vi "Test - Draw Teapot.vi"() -> ()   [LabVIEW 2022 SP3, in "Raster.lvlib"] (continued)
"v"=0.0}, "Colour"=12517256}, "Vertex 3"={"Position"={"x"=109.02176, "y"=274.10672, "z"=0.98959744}, "UV"={"u"=0.0, "v"=0.0}, "Colour"=12517256}, "Alpha"=0.0, "Alpha Blending Enabled"=FALSE, "Colour"=9684586}, {"Vertex 1"={"Position"={"x"=98.163345, "y"=283.49265, "z"=0.9895778}, "UV"={"u"=0.0, "v"=0.0}, "Colour"=12517256}, "Vertex 2"={"Position"={"x"=104.74968, "y"=271.31357, "z"=0.9895778}, "UV"={"u"=0.0, "v"=0.0}, "Colour"=12517256}, "Vertex 3"={"Position"={"x"=101.588585, "y"=268.6284, "z"=0.98959744}, "UV"={"u"=0.0, "v"=0.0}, "Colour"=12517256}, "Alpha"=0.0, "Alpha Blending Enabled"=FALSE, "Colour"=7773780}, {"Vertex 1"={"Position"={"x"=104.74968, "y"=271.31357, "z"=0.9895778}, "UV"={"u"=0.0, "v"=0.0}, "Colour"=12517256}, "Vertex 2"={"Position"={"x"=98.163345, "y"=283.49265, "z"=0.9895778}, "UV"={"u"=0.0, "v"=0.0}, "Colour"=12517256}, "Vertex 3"={"Position"={"x"=102.92444, "y"=285.8186, "z"=0.98959744}, "UV"={"u"=0.0, "v"=0.0}, "Colour"=12517256}, "Alpha"=0.0, "Alpha Blending Enabled"=FALSE, "Colour"=9486951}, {"Vertex 1"={"Position"={"x"=93.51947, "y"=295.5369, "z"=0.9895778}, "UV"={"u"=0.0, "v"=0.0}, "Colour"=12517256}, "Vertex 2"={"Position"={"x"=98.163345, "y"=283.49265, "z"=0.9895778}, "UV"={"u"=0.0, "v"=0.0}, "Colour"=12517256}, "Vertex 3"={"Position"={"x"=94.53805, "y"=281.22873, "z"=0.98959744}, "UV"={"u"=0.0, "v"=0.0}, "Colour"=12517256}, "Alpha"=0.0, "Alpha Blending Enabled"=FALSE, "Colour"=8037207}, {"Vertex 1"={"Position"={"x"=98.163345, "y"=283.49265, "z"=0.9895778}, "UV"={"u"=0.0, "v"=0.0}, "Colour"=12517256}, "Vertex 2"={"Position"={"x"=93.51947, "y"=295.5369, "z"=0.9895778}, "UV"={"u"=0.0, "v"=0.0}, "Colour"=12517256}, "Vertex 3"={"Position"={"x"=98.63565, "y"=297.2621, "z"=0.98959744}, "UV"={"u"=0.0, "v"=0.0}, "Colour"=12517256}, "Alpha"=0.0, "Alpha Blending Enabled"=FALSE, "Colour"=9289317}, {"Vertex 1"={"Position"={"x"=90.76903, "y"=307.28738, "z"=0.9895778}, "UV"={"u"=0.0, "v"=0.0}, "Colour"=12517256}, "Vertex 2"={"Position"={"x"=93.51947, "y"=295.5369, "z"=0.9895778}, "UV"={"u"=0.0, "v"=0.0}, "Colour"=12517256}, "Vertex 3"={"Position"={"x"=89.5565, "y"=293.82855, "z"=0.98959744}, "UV"={"u"=0.0, "v"=0.0}, "Colour"=12517256}, "Alpha"=0.0, "Alpha Blending Enabled"=FALSE, "Colour"=8300890}, {"Vertex 1"={"Position"={"x"=93.51947, "y"=295.5369, "z"=0.9895778}, "UV"={"u"=0.0, "v"=0.0}, "Colour"=12517256}, "Vertex 2"={"Position"={"x"=90.76903, "y"=307.28738, "z"=0.9895778}, "UV"={"u"=0.0, "v"=0.0}, "Colour"=12517256}, "Vertex 3"={"Position"={"x"=96.10178, "y"=308.23883, "z"=0.98959744}, "UV"={"u"=0.0, "v"=0.0}, "Colour"=12517256}, "Alpha"=0.0, "Alpha Blending Enabled"=FALSE, "Colour"=9091427}, {"Vertex 1"={"Position"={"x"=89.86314, "y"=318.58496, "z"=0.9895778}, "UV"={"u"=0.0, "v"=0.0}, "Colour"=12517256}, "Vertex 2"={"Position"={"x"=90.76903, "y"=307.28738, "z"=0.9895778}, "UV"={"u"=0.0, "v"=0.0}, "Colour"=12517256}, "Vertex 3"={"Position"={"x"=86.5999, "y"=306.30865, "z"=0.98959744}, "UV"={"u"=0.0, "v"=0.0}, "Colour"=12517256}, "Alpha"=0.0, "Alpha Blending Enabled"=FALSE, "Colour"=8564317}, {"Vertex 1"={"Position"={"x"=90.76903, "y"=307.28738, "z"=0.9895778}, "UV"={"u"=0.0, "v"=0.0}, "Colour"=12517256}, "Vertex 2"={"Position"={"x"=89.86314, "y"=318.58496, "z"=0.9895778}, "UV"={"u"=0.0, "v"=0.0}, "Colour"=12517256}, "Vertex 3"={"Position"={"x"=95.26916, "y"=318.55002, "z"=0.98959744}, "UV"={"u"=0.0, "v"=0.0}, "Colour"=12517256}, "Alpha"=0.0, "Alpha Blending Enabled"=FALSE, "Colour"=8828000}, {"Vertex 1"={"Position"={"x"=91.32674, "y"=328.538, "z"=0.9895778}, "UV"={"u"=0.0, "v"=0.0}, "Colour"=12517256}, "Vertex 2"={"Position"={"x"=89.86314, "y"=318.58496, "z"=0.9895778}, "UV"={"u"=0.0, "v"=0.0}, "Colour"=12517256}, "Vertex 3"={"Position"={"x"=85.62412, "y"=318.55002, "z"=0.98959744}, "UV"={"u"=0.0, "v"=0.0}, "Colour"=12517256}, "Alpha"=0.0, "Alpha Blending Enabled"=FALSE, "Colour"=8959585}, {"Vertex 1"={"Position"={"x"=89.86314, "y"=318.58496, "z"=0.9895778}, "UV"={"u"=0.0, "v"=0.0}, "Colour"=12517256}, "Vertex 2"={"Position"={"x"=91.32674, "y"=328.538, "z"=0.9895778}, "UV"={"u"=0.0, "v"=0.0}, "Colour"=12517256}, "Vertex 3"={"Position"={"x"=96.68016, "y"=327.50403, "z"=0.98959744}, "UV"={"u"=0.0, "v"=0.0}, "Colour"=12517256}, "Alpha"=0.0, "Alpha Blending Enabled"=FALSE, "Colour"=8432732}, {"Vertex 1"={"Position"={"x"=95.695854, "y"=336.50763, "z"=0.9895778}, "UV"={"u"=0.0, "v"=0.0}, "Colour"=12517256}, "Vertex 2"={"Position"={"x"=91.32674, "y"=328.538, "z"=0.9895778}, "UV"={"u"=0.0, "v"=0.0}, "Colour"=12517256}, "Vertex 3"={"Position"={"x"=87.13484, "y"=329.46445, "z"=0.98959744}, "UV"={"u"=0.0, "v"=0.0}, "Colour"=12517256}, "Alpha"=0.0, "Alpha Blending Enabled"=FALSE, "Colour"=9552488}, {"Vertex 1"={"Position"={"x"=91.32674, "y"=328.538, "z"=0.9895778}, "UV"={"u"=0.0, "v"=0.0}, "Colour"=12517256}, "Vertex 2"={"Position"={"x"=95.695854, "y"=336.50763, "z"=0.9895778}, "UV"={"u"=0.0, "v"=0.0}, "Colour"=12517256}, "Vertex 3"={"Position"={"x"=100.88518, "y"=334.67392, "z"=0.98959744}, "UV"={"u"=0.0, "v"=0.0}, "Colour"=12517256}, "Alpha"=0.0, "Alpha Blending Enabled"=FALSE, "Colour"=7839829}, {"Vertex 1"={"Position"={"x"=102.93782, "y"=342.71442, "z"=0.9895778}, "UV"={"u"=0.0, "v"=0.0}, "Colour"=12517256}, "Vertex 2"={"Position"={"x"=95.695854, "y"=336.50763, "z"=0.9895778}, "UV"={"u"=0.0, "v"=0.0}, "Colour"=12517256}, "Vertex 3"={"Position"={"x"=91.65158, "y"=338.20395, "z"=0.98959744}, "UV"={"u"=0.0, "v"=0.0}, "Colour"=12517256}, "Alpha"=0.0, "Alpha Blending Enabled"=FALSE, "Colour"=10079854}, {"Vertex 1"={"Position"={"x"=95.695854, "y"=336.50763, "z"=0.9895778}, "UV"={"u"=0.0, "v"=0.0}, "Colour"=12517256}, "Vertex 2"={"Position"={"x"=102.93782, "y"=342.71442, "z"=0.9895778}, "UV"={"u"=0.0, "v"=0.0}, "Colour"=12517256}, "Vertex 3"={"Position"={"x"=107.84178, "y"=340.25775, "z"=0.98959744}, "UV"={"u"=0.0, "v"=0.0}, "Colour"=12517256}, "Alpha"=0.0, "Alpha Blending Enabled"=FALSE, "Colour"=7246927}, {"Vertex 1"={"Position"={"x"=113.01999, "y"=347.37875, "z"=0.9895778}, "UV"={"u"=0.0, "v"=0.0}, "Colour"=12517256}, "Vertex 2"={"Position"={"x"=102.93782, "y"=342.71442, "z"=0.9895778}, "UV"={"u"=0.0, "v"=0.0}, "Colour"=12517256}, "Vertex 3"={"Position"={"x"=99.15168, "y"=345.0104, "z"=0.98959744}, "UV"={"u"=0.0, "v"=0.0}, "Colour"=12517256}, "Alpha"=0.0, "Alpha Blending Enabled"=FALSE, "Colour"=10540658}, {"Vertex 1"={"Position"={"x"=102.93782, "y"=342.71442, "z"=0.9895778}, "UV"={"u"=0.0, "v"=0.0}, "Colour"=12517256}, "Vertex 2"={"Position"={"x"=113.01999, "y"=347.37875, "z"=0.9895778}, "UV"={"u"=0.0, "v"=0.0}, "Colour"=12517256}, "Vertex 3"={"Position"={"x"=117.50798, "y"=344.45398, "z"=0.98959744}, "UV"={"u"=0.0, "v"=0.0}, "Colour"=12517256}, "Alpha"=0.0, "Alpha Blending Enabled"=FALSE, "Colour"=6785866}, {"Vertex 1"={"Position"={"x"=125.90974, "y"=350.72086, "z"=0.9895778}, "UV"={"u"=0.0, "v"=0.0}, "Colour"=12517256}, "Vertex 2"={"Position"={"x"=113.01999, "y"=347.37875, "z"=0.9895778}, "UV"={"u"=0.0, "v"=0.0}, "Colour"=12517256}, "Vertex 3"={"Position"={"x"=109.61189, "y"=350.12524, "z"=0.98959744}, "UV"={"u"=0.0, "v"=0.0}, "Colour"=12517256}, "Alpha"=0.0, "Alpha Blending Enabled"=FALSE, "Colour"=10738549}, {"Vertex 1"={"Position"={"x"=113.01999, "y"=347.37875, "z"=0.9895778}, "UV"={"u"=0.0, "v"=0.0}, "Colour"=12517256}, "Vertex 2"={"Position"={"x"=125.90974, "y"=350.72086, "z"=0.9895778}, "UV"={"u"=0.0, "v"=0.0}, "Colour"=12517256}, "Vertex 3"={"Position"={"x"=129.84137, "y"=347.46066, "z"=0.98959744}, "UV"={"u"=0.0, "v"=0.0}, "Colour"=12517256}, "Alpha"=0.0, "Alpha Blending Enabled"=FALSE, "Colour"=6522183}, {"Vertex 1"={"Position"={"x"=141.57439, "y"=352.9612, "z"=0.9895778}, "UV"={"u"=0.0, "v"=0.0}, "Colour"=12517256}, "Vertex 2"={"Position"={"x"=125.90974, "y"=350.72086, "z"=0.9895778}, "UV"={"u"=0.0, "v"=0.0}, "Colour"=12517256}, "Vertex 3"={"Position"={"x"=123.00947, "y"=353.7902, "z"=0.98959744}, "UV"={"u"=0.0, "v"=0.0}, "Colour"=12517256}, "Alpha"=0.0, "Alpha Blending Enabled"=FALSE, "Colour"=10804598}, {"Vertex 1"={"Position"={"x"=125.90974, "y"=350.72086, "z"=0.9895778}, "UV"={"u"=0.0, "v"=0.0}, "Colour"=12517256}, "Vertex 2"={"Position"={"x"=141.57439, "y"=352.9612, "z"=0.9895778}, "UV"={"u"=0.0, "v"=0.0}, "Colour"=12517256}, "Vertex 3"={"Position"={"x"=144.79973, "y"=349.47617, "z"=0.98959744}, "UV"={"u"=0.0, "v"=0.0}, "Colour"=12517256}, "Alpha"=0.0, "Alpha Blending Enabled"=FALSE, "Colour"=6324549}, {"Vertex 1"={"Position"={"x"=159.98125, "y"=354.3201, "z"=0.9895778}, "UV"={"u"=0.0, "v"=0.0}, "Colour"=12517256}, "Vertex 2"={"Position"={"x"=141.57439, "y"=352.9612, "z"=0.9895778}, "UV"={"u"=0.0, "v"=0.0}, "Colour"=12517256}, "Vertex 3"={"Position"={"x"=139.3214, "y"=356.247, "z"=0.98959744}, "UV"={"u"=0.0, "v"=0.0}, "Colour"=12517256}, "Alpha"=0.0, "Alpha Blending Enabled"=FALSE, "Colour"=10870134}, {"Vertex 1"={"Position"={"x"=141.57439, "y"=352.9612, "z"=0.9895778}, "UV"={"u"=0.0, "v"=0.0}, "Colour"=12517256}, "Vertex 2"={"Position"={"x"=159.98125, "y"=354.3201, "z"=0.9895778}, "UV"={"u"=0.0, "v"=0.0}, "Colour"=12517256}, "Vertex 3"={"Position"={"x"=162.341, "y"=350.69873, "z"=0.98959744}, "UV"={"u"=0.0, "v"=0.0}, "Colour"=12517256}, "Alpha"=0.0, "Alpha Blending Enabled"=FALSE, "Colour"=6258756}, {"Vertex 1"={"Position"={"x"=181.09776, "y"=355.0179, "z"=0.9895778}, "UV"={"u"=0.0, "v"=0.0}, "Colour"=12517256}, "Vertex 2"={"Position"={"x"=159.98125, "y"=354.3201, "z"=0.9895778}, "UV"={"u"=0.0, "v"=0.0}, "Colour"=12517256}, "Vertex 3"={"Position"={"x"=158.52467, "y"=357.73706, "z"=0.98959744}, "UV"={"u"=0.0, "v"=0.0}, "Colour"=12517256}, "Alpha"=0.0, "Alpha Blending Enabled"=FALSE, "Colour"=10870134}, {"Vertex 1"={"Position"={"x"=159.98125, "y"=354.3201, "z"=0.9895778}, "UV"={"u"=0.0, "v"=0.0}, "Colour"=12517256}, "Vertex 2"={"Position"={"x"=181.09776, "y"=355.0179, "z"=0.9895778}, "UV"={"u"=0.0, "v"=0.0}, "Colour"=12517256}, "Vertex 3"={"Position"={"x"=182.42264, "y"=351.32635, "z"=0.98959744}, "UV"={"u"=0.0, "v"=0.0}, "Colour"=12517256}, "Alpha"=0.0, "Alpha Blending Enabled"=FALSE, "Colour"=6258500}, {"Vertex 1"={"Position"={"x"=204.89125, "y"=355.27502, "z"=0.9895778}, "UV"={"u"=0.0, "v"=0.0}, "Colour"=12517256}, "Vertex 2"={"Position"={"x"=181.09776, "y"=355.0179, "z"=0.9895778}, "UV"={"u"=0.0, "v"=0.0}, "Colour"=12517256}, "Vertex 3"={"Position"={"x"=180.59659, "y"=358.50238, "z"=0.98959744}, "UV"={"u"=0.0, "v"=0.0}, "Colour"=12517256}, "Alpha"=0.0, "Alpha Blending Enabled"=FALSE, "Colour"=10870134}, {"Vertex 1"={"Position"={"x"=181.09776, "y"=355.0179, "z"=0.9895778}, "UV"={"u"=0.0, "v"=0.0}, "Colour"=12517256}, "Vertex 2"={"Position"={"x"=204.89125, "y"=355.27502, "z"=0.9895778}, "UV"={"u"=0.0, "v"=0.0}, "Colour"=12517256}, "Vertex 3"={"Position"={"x"=205.00276, "y"=351.5577, "z"=0.98959744}, "UV"={"u"=0.0, "v"=0.0}, "Colour"=12517256}, "Alpha"=0.0, "Alpha Blending Enabled"=FALSE, "Colour"=6258500}, {"Vertex 1"={"Position"={"x"=231.32906, "y"=355.31174, "z"=0.9895778}, "UV"={"u"=0.0, "v"=0.0}, "Colour"=12517256}, "Vertex 2"={"Position"={"x"=204.89125, "y"=355.27502, "z"=0.9895778}, "UV"={"u"=0.0, "v"=0.0}, "Colour"=12517256}, "Vertex 3"={"Position"={"x"=205.5139, "y"=358.7842, "z"=0.98959744}, "UV"={"u"=0.0, "v"=0.0}, "Colour"=12517256}, "Alpha"=0.0, "Alpha Blending Enabled"=FALSE, "Colour"=10870134}, {"Vertex 1"={"Position"={"x"=204.89125, "y"=355.27502, "z"=0.9895778}, "UV"={"u"=0.0, "v"=0.0}, "Colour"=12517256}, "Vertex 2"={"Position"={"x"=231.32906, "y"=355.31174, "z"=0.9895778}, "UV"={"u"=0.0, "v"=0.0}, "Colour"=12517256}, "Vertex 3"={"Position"={"x"=230.03891, "y"=351.59073, "z"=0.98959744}, "UV"={"u"=0.0, "v"=0.0}, "Colour"=12517256}, "Alpha"=0.0, "Alpha Blending Enabled"=FALSE, "Colour"=6258500}, {"Vertex 1"={"Position"={"x"=583.19836, "y"=275.50385, "z"=0.9896794}, "UV"={"u"=0.0, "v"=0.0}, "Colour"=12517256}, "Vertex 2"={"Position"={"x"=608.8621, "y"=277.8157, "z"=0.9896861}, "UV"={"u"=0.0, "v"=0.0}, "Colour"=12517256}, "Vertex 3"={"Position"={"x"=615.98, "y"=270.86078, "z"=0.989385}, "UV"={"u"=0.0, "v"=0.0}, "Colour"=12517256}, "Alpha"=0.0, "Alpha Blending Enabled"=FALSE, "Colour"=11594878}, {"Vertex 1"={"Position"={"x"=689.394, "y"=356.5748, "z"=0.98960906}, "UV"={"u"=0.0, "v"=0.0}, "Colour"=12517256}, "Vertex 2"={"Position"={"x"=683.931, "y"=340.25684, "z"=0.98953646}, "UV"={"u"=0.0, "v"=0.0}, "Colour"=12517256}, "Vertex 3"={"Position"={"x"=677.0391, "y"=342.4919, "z"=0.9896034}, "UV"={"u"=0.0, "v"=0.0}, "Colour"=12517256}, "Alpha"=0.0, "Alpha Blending Enabled"=FALSE, "Colour"=10672756}, {"Vertex 1"={"Position"={"x"=180.41942, "y"=218.89479, "z"=0.9893465}, "UV"={"u"=0.0, "v"=0.0}, "Colour"=12517256}, "Vertex 2"={"Position"={"x"=182.0637, "y"=204.669, "z"=0.98935175}, "UV"={"u"=0.0, "v"=0.0}, "Colour"=12517256}, "Vertex 3"={"Position"={"x"=193.60881, "y"=210.88196, "z"=0.990049}, "UV"={"u"=0.0, "v"=0.0}, "Colour"=12517256}, "Alpha"=0.0, "Alpha Blending Enabled"=FALSE, "Colour"=131841}, {"Vertex 1"={"Position"={"x"=617.93634, "y"=204.669, "z"=0.98935175}, "UV"={"u"=0.0, "v"=0.0}, "Colour"=12517256}, "Vertex 2"={"Position"={"x"=619.58057, "y"=218.89479, "z"=0.9893465}, "UV"={"u"=0.0, "v"=0.0}, "Colour"=12517256}, "Vertex 3"={"Position"={"x"=607.8461, "y"=224.21788, "z"=0.990049}, "UV"={"u"=0.0, "v"=0.0}, "Colour"=12517256}, "Alpha"=0.0, "Alpha Blending Enabled"=FALSE, "Colour"=131841}, {"Vertex 1"={"Position"={"x"=181.27118, "y"=234.16856, "z"=0.98934925}, "UV"={"u"=0.0, "v"=0.0}, "Colour"=12517256}, "Vertex 2"={"Position"={"x"=180.41942, "y"=218.89479, "z"=0.9893465}, "UV"={"u"=0.0, "v"=0.0}, "Colour"=12517256}, "Vertex 3"={"Position"={"x"=192.15388, "y"=224.21788, "z"=0.990049}, "UV"={"u"=0.0, "v"=0.0}, "Colour"=12517256}, "Alpha"=0.0, "Alpha Blending Enabled"=FALSE, "Colour"=1185805}, {"Vertex 1"={"Position"={"x"=619.58057, "y"=218.89479, "z"=0.9893465}, "UV"={"u"=0.0, "v"=0.0}, "Colour"=12517256}, "Vertex 2"={"Position"={"x"=618.7288, "y"=234.16856, "z"=0.98934925}, "UV"={"u"=0.0, "v"=0.0}, "Colour"=12517256}, "Vertex 3"={"Position"={"x"=607.09265, "y"=238.47354, "z"=0.990049}, "UV"={"u"=0.0, "v"=0.0}, "Colour"=12517256}, "Alpha"=0.0, "Alpha Blending Enabled"=FALSE, "Colour"=1185805}, {"Vertex 1"={"Position"={"x"=389.09088, "y"=464.3185, "z"=0.98942566}, "UV"={"u"=0.0, "v"=0.0}, "Colour"=12517256}, "Vertex 2"={"Position"={"x"=393.28003, "y"=463.19003, "z"=0.98966503}, "UV"={"u"=0.0, "v"=0.0}, "Colour"=12517256}, "Vertex 3"={"Position"={"x"=396.5364, "y"=463.4357, "z"=0.9896494}, "UV"={"u"=0.0, "v"=0.0}, "Colour"=12517256}, "Alpha"=0.0, "Alpha Blending Enabled"=FALSE, "Colour"=10409073}, {"Vertex 1"={"Position"={"x"=621.5498, "y"=201.64421, "z"=0.9896861}, "UV"={"u"=0.0, "v"=0.0}, "Colour"=12517256}, "Vertex 2"={"Position"={"x"=583.19836, "y"=191.57744, "z"=0.9896794}, "UV"={"u"=0.0, "v"=0.0}, "Colour"=12517256}, "Vertex 3"={"Position"={"x"=588.6202, "y"=195.32538, "z"=0.9893725}, "UV"={"u"=0.0, "v"=0.0}, "Colour"=12517256}, "Alpha"=0.0, "Alpha Blending Enabled"=FALSE, "Colour"=131841}, {"Vertex 1"={"Position"={"x"=683.931, "y"=340.25684, "z"=0.98953646}, "UV"={"u"=0.0, "v"=0.0}, "Colour"=12517256}, "Vertex 2"={"Position"={"x"=689.394, "y"=356.5748, "z"=0.98960906}, "UV"={"u"=0.0, "v"=0.0}, "Colour"=12517256}, "Vertex 3"={"Position"={"x"=696.25714, "y"=355.18262, "z"=0.98958987}, "UV"={"u"=0.0, "v"=0.0}, "Colour"=12517256}, "Alpha"=0.0, "Alpha Blending Enabled"=FALSE, "Colour"=10738549}, {"Vertex 1"={"Position"={"x"=394.9576, "y"=413.28833, "z"=0.9894651}, "UV"={"u"=0.0, "v"=0.0}, "Colour"=12517256}, "Vertex 2"={"Position"={"x"=396.44946, "y"=415.85388, "z"=0.98963785}, "UV"={"u"=0.0, "v"=0.0}, "Colour"=12517256}, "Vertex 3"={"Position"={"x"=400.0, "y"=415.91602, "z"=0.9896323}, "UV"={"u"=0.0, "v"=0.0}, "Colour"=12517256}, "Alpha"=0.0, "Alpha Blending Enabled"=FALSE, "Colour"=11924353}, {"Vertex 1"={"Position"={"x"=400.0, "y"=130.68715, "z"=0.990049}, "UV"={"u"=0.0, "v"=0.0}, "Colour"=12517256}, "Vertex 2"={"Position"={"x"=374.42786, "y"=119.574394, "z"=0.98937833}, "UV"={"u"=0.0, "v"=0.0}, "Colour"=12517256}, "Vertex 3"={"Position"={"x"=379.93253, "y"=118.36189, "z"=0.9893066}, "UV"={"u"=0.0, "v"=0.0}, "Colour"=12517256}, "Alpha"=0.0, "Alpha Blending Enabled"=FALSE, "Colour"=131841}, {"Vertex 1"={"Position"={"x"=400.0, "y"=130.68715, "z"=0.990049}, "UV"={"u"=0.0, "v"=0.0}, "Colour"=12517256}, "Vertex 2"={"Position"={"x"=420.06744, "y"=118.36189, "z"=0.9893066}, "UV"={"u"=0.0, "v"=0.0}, "Colour"=12517256}, "Vertex 3"={"Position"={"x"=425.57214, "y"=119.574394, "z"=0.98937833}, "UV"={"u"=0.0, "v"=0.0}, "Colour"=12517256}, "Alpha"=0.0, "Alpha Blending Enabled"=FALSE, "Colour"=131841}, {"Vertex 1"={"Position"={"x"=424.30502, "y"=410.7137, "z"=0.9897057}, "UV"={"u"=0.0, "v"=0.0}, "Colour"=12517256}, "Vertex 2"={"Position"={"x"=434.50436, "y"=408.5937, "z"=0.9895617}, "UV"={"u"=0.0, "v"=0.0}, "Colour"=12517256}, "Vertex 3"={"Position"={"x"=430.5626, "y"=409.63797, "z"=0.98946077}, "UV"={"u"=0.0, "v"=0.0}, "Colour"=12517256}, "Alpha"=0.0, "Alpha Blending Enabled"=FALSE, "Colour"=10145390}, {"Vertex 1"={"Position"={"x"=657.4915, "y"=300.53033, "z"=0.9895282}, "UV"={"u"=0.0, "v"=0.0}, "Colour"=12517256}, "Vertex 2"={"Position"={"x"=648.9251, "y"=288.04398, "z"=0.9894685}, "UV"={"u"=0.0, "v"=0.0}, "Colour"=12517256}, "Vertex 3"={"Position"={"x"=640.6776, "y"=292.91815, "z"=0.9897306}, "UV"={"u"=0.0, "v"=0.0}, "Colour"=12517256}, "Alpha"=0.0, "Alpha Blending Enabled"=FALSE, "Colour"=8630366}, {"Vertex 1"={"Position"={"x"=400.0, "y"=413.3747, "z"=0.9894571}, "UV"={"u"=0.0, "v"=0.0}, "Colour"=12517256}, "Vertex 2"={"Position"={"x"=400.0, "y"=415.91602, "z"=0.9896323}, "UV"={"u"=0.0, "v"=0.0}, "Colour"=12517256}, "Vertex 3"={"Position"={"x"=403.55054, "y"=415.85388, "z"=0.98963785}, "UV"={"u"=0.0, "v"=0.0}, "Colour"=12517256}, "Alpha"=0.0, "Alpha Blending Enabled"=FALSE, "Colour"=11924353}, {"Vertex 1"={"Position"={"x"=360.7029, "y"=126.617645, "z"=0.98979497}, "UV"={"u"=0.0, "v"=0.0}, "Colour"=12517256}, "Vertex 2"={"Position"={"x"=327.3322, "y"=123.64719, "z"=0.9895792}, "UV"={"u"=0.0, "v"=0.0}, "Colour"=12517256}, "Vertex 3"={"Position"={"x"=330.4428, "y"=119.82906, "z"=0.98935246}, "UV"={"u"=0.0, "v"=0.0}, "Colour"=12517256}, "Alpha"=0.0, "Alpha Blending Enabled"=FALSE, "Colour"=131841}, {"Vertex 1"={"Position"={"x"=372.0999, "y"=453.91602, "z"=0.98951197}, "UV"={"u"=0.0, "v"=0.0}, "Colour"=12517256}, "Vertex 2"={"Position"={"x"=374.82742, "y"=447.3146, "z"=0.98956454}, "UV"={"u"=0.0, "v"=0.0}, "Colour"=12517256}, "Vertex 3"={"Position"={"x"=371.54373, "y"=446.1597, "z"=0.9896467}, "UV"={"u"=0.0, "v"=0.0}, "Colour"=12517256}, "Alpha"=0.0, "Alpha Blending Enabled"=FALSE, "Colour"=197634}, {"Vertex 1"={"Position"={"x"=378.79004, "y"=448.31607, "z"=0.98949325}, "UV"={"u"=0.0, "v"=0.0}, "Colour"=12517256}, "Vertex 2"={"Position"={"x"=382.30276, "y"=440.7109, "z"=0.9895852}, "UV"={"u"=0.0, "v"=0.0}, "Colour"=12517256}, "Vertex 3"={"Position"={"x"=378.97202, "y"=439.917, "z"=0.9896443}, "UV"={"u"=0.0, "v"=0.0}, "Colour"=12517256}, "Alpha"=0.0, "Alpha Blending Enabled"=FALSE, "Colour"=131841}, {"Vertex 1"={"Position"={"x"=368.48776, "y"=452.57986, "z"=0.9896035}, "UV"={"u"=0.0, "v"=0.0}, "Colour"=12517256}, "Vertex 2"={"Position"={"x"=368.50552, "y"=457.60767, "z"=0.98960376}, "UV"={"u"=0.0, "v"=0.0}, "Colour"=12517256}, "Vertex 3"={"Position"={"x"=372.1155, "y"=458.98697, "z"=0.9895123}, "UV"={"u"=0.0, "v"=0.0}, "Colour"=12517256}, "Alpha"=0.0, "Alpha Blending Enabled"=FALSE, "Colour"=5797439}, {"Vertex 1"={"Position"={"x"=431.49448, "y"=457.60767, "z"=0.98960376}, "UV"={"u"=0.0, "v"=0.0}, "Colour"=12517256}, "Vertex 2"={"Position"={"x"=431.51227, "y"=452.57986, "z"=0.9896035}, "UV"={"u"=0.0, "v"=0.0}, "Colour"=12517256}, "Vertex 3"={"Position"={"x"=427.9001, "y"=453.91602, "z"=0.98951197}, "UV"={"u"=0.0, "v"=0.0}, "Colour"=12517256}, "Alpha"=0.0, "Alpha Blending Enabled"=FALSE, "Colour"=5797439}, {"Vertex 1"={"Position"={"x"=405.62814, "y"=464.7204, "z"=0.9893997}, "UV"={"u"=0.0, "v"=0.0}, "Colour"=12517256}, "Vertex 2"={"Position"={"x"=403.4636, "y"=463.4357, "z"=0.9896494}, "UV"={"u"=0.0, "v"=0.0}, "Colour"=12517256}, "Vertex 3"={"Position"={"x"=406.71997, "y"=463.19003, "z"=0.98966503}, "UV"={"u"=0.0, "v"=0.0}, "Colour"=12517256}, "Alpha"=0.0, "Alpha Blending Enabled"=FALSE, "Colour"=10409073}, {"Vertex 1"={"Position"={"x"=412.42462, "y"=462.27194, "z"=0.98972344}, "UV"={"u"=0.0, "v"=0.0}, "Colour"=12517256}, "Vertex 2"={"Position"={"x"=420.0997, "y"=462.82288, "z"=0.98952234}, "UV"={"u"=0.0, "v"=0.0}, "Colour"=12517256}, "Vertex 3"={"Position"={"x"=415.7588, "y"=463.67755, "z"=0.98946714}, "UV"={"u"=0.0, "v"=0.0}, "Colour"=12517256}, "Alpha"=0.0, "Alpha Blending Enabled"=FALSE, "Colour"=10211439}, {"Vertex 1"={"Position"={"x"=690.1191, "y"=337.60867, "z"=0.98951393}, "UV"={"u"=0.0, "v"=0.0}, "Colour"=12517256}, "Vertex 2"={"Position"={"x"=696.25714, "y"=355.18262, "z"=0.98958987}, "UV"={"u"=0.0, "v"=0.0}, "Colour"=12517256}, "Vertex 3"={"Position"={"x"=702.0343, "y"=353.5881, "z"=0.98960906}, "UV"={"u"=0.0, "v"=0.0}, "Colour"=12517256}, "Alpha"=0.0, "Alpha Blending Enabled"=FALSE, "Colour"=9750122}, {"Vertex 1"={"Position"={"x"=409.59305, "y"=441.8486, "z"=0.98950064}, "UV"={"u"=0.0, "v"=0.0}, "Colour"=12517256}, "Vertex 2"={"Position"={"x"=407.6209, "y"=433.84442, "z"=0.9896132}, "UV"={"u"=0.0, "v"=0.0}, "Colour"=12517256}, "Vertex 3"={"Position"={"x"=403.92798, "y"=434.0735, "z"=0.9895953}, "UV"={"u"=0.0, "v"=0.0}, "Colour"=12517256}, "Alpha"=0.0, "Alpha Blending Enabled"=FALSE, "Colour"=461317}, {"Vertex 1"={"Position"={"x"=472.6678, "y"=123.64719, "z"=0.9895792}, "UV"={"u"=0.0, "v"=0.0}, "Colour"=12517256}, "Vertex 2"={"Position"={"x"=500.08884, "y"=121.74838, "z"=0.98940194}, "UV"={"u"=0.0, "v"=0.0}, "Colour"=12517256}, "Vertex 3"={"Position"={"x"=500.85635, "y"=127.179695, "z"=0.98972636}, "UV"={"u"=0.0, "v"=0.0}, "Colour"=12517256}, "Alpha"=0.0, "Alpha Blending Enabled"=FALSE, "Colour"=131841}, {"Vertex 1"={"Position"={"x"=376.1374, "y"=461.78098, "z"=0.98958975}, "UV"={"u"=0.0, "v"=0.0}, "Colour"=12517256}, "Vertex 2"={"Position"={"x"=372.1155, "y"=458.98697, "z"=0.9895123}, "UV"={"u"=0.0, "v"=0.0}, "Colour"=12517256}, "Vertex 3"={"Position"={"x"=368.50552, "y"=457.60767, "z"=0.98960376}, "UV"={"u"=0.0, "v"=0.0}, "Colour"=12517256}, "Alpha"=0.0, "Alpha Blending Enabled"=FALSE, "Colour"=10540914}, {"Vertex 1"={"Position"={"x"=378.97202, "y"=439.917, "z"=0.9896443}, "UV"={"u"=0.0, "v"=0.0}, "Colour"=12517256}, "Vertex 2"={"Position"={"x"=374.82742, "y"=447.3146, "z"=0.98956454}, "UV"={"u"=0.0, "v"=0.0}, "Colour"=12517256}, "Vertex 3"={"Position"={"x"=378.79004, "y"=448.31607, "z"=0.98949325}, "UV"={"u"=0.0, "v"=0.0}, "Colour"=12517256}, "Alpha"=0.0, "Alpha Blending Enabled"=FALSE, "Colour"=131841}, {"Vertex 1"={"Position"={"x"=409.97757, "y"=415.3864, "z"=0.9896799}, "UV"={"u"=0.0, "v"=0.0}, "Colour"=12517256}, "Vertex 2"={"Position"={"x"=414.14594, "y"=412.64026, "z"=0.98952574}, "UV"={"u"=0.0, "v"=0.0}, "Colour"=12517256}, "Vertex 3"={"Position"={"x"=409.7829, "y"=413.03857, "z"=0.9894885}, "UV"={"u"=0.0, "v"=0.0}, "Colour"=12517256}, "Alpha"=0.0, "Alpha Blending Enabled"=FALSE, "Colour"=11594878}, {"Vertex 1"={"Position"={"x"=394.37186, "y"=464.7204, "z"=0.9893997}, "UV"={"u"=0.0, "v"=0.0}, "Colour"=12517256}, "Vertex 2"={"Position"={"x"=396.5364, "y"=463.4357, "z"=0.9896494}, "UV"={"u"=0.0, "v"=0.0}, "Colour"=12517256}, "Vertex 3"={"Position"={"x"=400.0, "y"=463.52048, "z"=0.98964405}, "UV"={"u"=0.0, "v"=0.0}, "Colour"=12517256}, "Alpha"=0.0, "Alpha Blending Enabled"=FALSE, "Colour"=10474866}, {"Vertex 1"={"Position"={"x"=502.8223, "y"=396.39102, "z"=0.98972005}, "UV"={"u"=0.0, "v"=0.0}, "Colour"=12517256}, "Vertex 2"={"Position"={"x"=517.09094, "y"=394.1647, "z"=0.98967445}, "UV"={"u"=0.0, "v"=0.0}, "Colour"=12517256}, "Vertex 3"={"Position"={"x"=516.79083, "y"=397.61792, "z"=0.98929393}, "UV"={"u"=0.0, "v"=0.0}, "Colour"=12517256}, "Alpha"=0.0, "Alpha Blending Enabled"=FALSE, "Colour"=9091427}, {"Vertex 1"={"Position"={"x"=693.6034, "y"=307.21713, "z"=0.9896555}, "UV"={"u"=0.0, "v"=0.0}, "Colour"=12517256}, "Vertex 2"={"Position"={"x"=688.6595, "y"=283.87192, "z"=0.9895922}, "UV"={"u"=0.0, "v"=0.0}, "Colour"=12517256}, "Vertex 3"={"Position"={"x"=689.1351, "y"=288.03708, "z"=0.9894408}, "UV"={"u"=0.0, "v"=0.0}, "Colour"=12517256}, "Alpha"=0.0, "Alpha Blending Enabled"=FALSE, "Colour"=3030561}, {"Vertex 1"={"Position"={"x"=395.05292, "y"=442.15393, "z"=0.98947793}, "UV"={"u"=0.0, "v"=0.0}, "Colour"=12517256}, "Vertex 2"={"Position"={"x"=396.07202, "y"=434.0735, "z"=0.9895953}, "UV"={"u"=0.0, "v"=0.0}, "Colour"=12517256}, "Vertex 3"={"Position"={"x"=392.3791, "y"=433.84442, "z"=0.9896132}, "UV"={"u"=0.0, "v"=0.0}, "Colour"=12517256}, "Alpha"=0.0, "Alpha Blending Enabled"=FALSE, "Colour"=461317}, {"Vertex 1"={"Position"={"x"=453.6991, "y"=404.1098, "z"=0.98970187}, "UV"={"u"=0.0, "v"=0.0}, "Colour"=12517256}, "Vertex 2"={"Position"={"x"=469.47156, "y"=402.4644, "z"=0.9895999}, "UV"={"u"=0.0, "v"=0.0}, "Colour"=12517256}, "Vertex 3"={"Position"={"x"=466.43457, "y"=404.58322, "z"=0.98938376}, "UV"={"u"=0.0, "v"=0.0}, "Colour"=12517256}, "Alpha"=0.0, "Alpha Blending Enabled"=FALSE, "Colour"=9289061}, {"Vertex 1"={"Position"={"x"=400.0, "y"=464.85934, "z"=0.98939073}, "UV"={"u"=0.0, "v"=0.0}, "Colour"=12517256}, "Vertex 2"={"Position"={"x"=400.0, "y"=463.52048, "z"=0.98964405}, "UV"={"u"=0.0, "v"=0.0}, "Colour"=12517256}, "Vertex 3"={"Position"={"x"=403.4636, "y"=463.4357, "z"=0.9896494}, "UV"={"u"=0.0, "v"=0.0}, "Colour"=12517256}, "Alpha"=0.0, "Alpha Blending Enabled"=FALSE, "Colour"=10474866}, {"Vertex 1"={"Position"={"x"=425.17258, "y"=447.3146, "z"=0.98956454}, "UV"={"u"=0.0, "v"=0.0}, "Colour"=12517256}, "Vertex 2"={"Position"={"x"=427.9001, "y"=453.91602, "z"=0.98951197}, "UV"={"u"=0.0, "v"=0.0}, "Colour"=12517256}, "Vertex 3"={"Position"={"x"=431.51227, "y"=452.57986, "z"=0.9896035}, "UV"={"u"=0.0, "v"=0.0}, "Colour"=12517256}, "Alpha"=0.0, "Alpha Blending Enabled"=FALSE, "Colour"=197634}, {"Vertex 1"={"Position"={"x"=388.97626, "y"=433.47845, "z"=0.9896417}, "UV"={"u"=0.0, "v"=0.0}, "Colour"=12517256}, "Vertex 2"={"Position"={"x"=386.13464, "y"=441.3613, "z"=0.9895369}, "UV"={"u"=0.0, "v"=0.0}, "Colour"=12517256}, "Vertex 3"={"Position"={"x"=390.40692, "y"=441.8486, "z"=0.98950064}, "UV"={"u"=0.0, "v"=0.0}, "Colour"=12517256}, "Alpha"=0.0, "Alpha Blending Enabled"=FALSE, "Colour"=131842}, {"Vertex 1"={"Position"={"x"=390.27826, "y"=462.79736, "z"=0.98969}, "UV"={"u"=0.0, "v"=0.0}, "Colour"=12517256}, "Vertex 2"={"Position"={"x"=384.2412, "y"=463.67755, "z"=0.98946714}, "UV"={"u"=0.0, "v"=0.0}, "Colour"=12517256}, "Vertex 3"={"Position"={"x"=379.9003, "y"=462.82288, "z"=0.98952234}, "UV"={"u"=0.0, "v"=0.0}, "Colour"=12517256}, "Alpha"=0.0, "Alpha Blending Enabled"=FALSE, "Colour"=10211439}, {"Vertex 1"={"Position"={"x"=369.4374, "y"=409.63797, "z"=0.98946077}, "UV"={"u"=0.0, "v"=0.0}, "Colour"=12517256}, "Vertex 2"={"Position"={"x"=378.53265, "y"=411.46152, "z"=0.9896358}, "UV"={"u"=0.0, "v"=0.0}, "Colour"=12517256}, "Vertex 3"={"Position"={"x"=381.9381, "y"=412.10922, "z"=0.98957527}, "UV"={"u"=0.0, "v"=0.0}, "Colour"=12517256}, "Alpha"=0.0, "Alpha Blending Enabled"=FALSE, "Colour"=10409073}, {"Vertex 1"={"Position"={"x"=393.107, "y"=415.6739, "z"=0.98965406}, "UV"={"u"=0.0, "v"=0.0}, "Colour"=12517256}, "Vertex 2"={"Position"={"x"=390.2171, "y"=413.03857, "z"=0.9894885}, "UV"={"u"=0.0, "v"=0.0}, "Colour"=12517256}, "Vertex 3"={"Position"={"x"=385.85406, "y"=412.64026, "z"=0.98952574}, "UV"={"u"=0.0, "v"=0.0}, "Colour"=12517256}, "Alpha"=0.0, "Alpha Blending Enabled"=FALSE, "Colour"=11594878}, {"Vertex 1"={"Position"={"x"=673.70026, "y"=326.4925, "z"=0.98952615}, "UV"={"u"=0.0, "v"=0.0}, "Colour"=12517256}, "Vertex 2"={"Position"={"x"=677.0391, "y"=342.4919, "z"=0.9896034}, "UV"={"u"=0.0, "v"=0.0}, "Colour"=12517256}, "Vertex 3"={"Position"={"x"=683.931, "y"=340.25684, "z"=0.98953646}, "UV"={"u"=0.0, "v"=0.0}, "Colour"=12517256}, "Alpha"=0.0, "Alpha Blending Enabled"=FALSE, "Colour"=10540658}, {"Vertex 1"={"Position"={"x"=404.94708, "y"=442.15393, "z"=0.98947793}, "UV"={"u"=0.0, "v"=0.0}, "Colour"=12517256}, "Vertex 2"={"Position"={"x"=403.92798, "y"=434.0735, "z"=0.9895953}, "UV"={"u"=0.0, "v"=0.0}, "Colour"=12517256}, "Vertex 3"={"Position"={"x"=400.0, "y"=434.1526, "z"=0.9895892}, "UV"={"u"=0.0, "v"=0.0}, "Colour"=12517256}, "Alpha"=0.0, "Alpha Blending Enabled"=FALSE, "Colour"=658951}, {"Vertex 1"={"Position"={"x"=702.0343, "y"=353.5881, "z"=0.98960906}, "UV"={"u"=0.0, "v"=0.0}, "Colour"=12517256}, "Vertex 2"={"Position"={"x"=695.06805, "y"=334.79984, "z"=0.98953646}, "UV"={"u"=0.0, "v"=0.0}, "Colour"=12517256}, "Vertex 3"={"Position"={"x"=690.1191, "y"=337.60867, "z"=0.98951393}, "UV"={"u"=0.0, "v"=0.0}, "Colour"=12517256}, "Alpha"=0.0, "Alpha Blending Enabled"=FALSE, "Colour"=9223268}, {"Vertex 1"={"Position"={"x"=378.53265, "y"=411.46152, "z"=0.9896358}, "UV"={"u"=0.0, "v"=0.0}, "Colour"=12517256}, "Vertex 2"={"Position"={"x"=369.4374, "y"=409.63797, "z"=0.98946077}, "UV"={"u"=0.0, "v"=0.0}, "Colour"=12517256}, "Vertex 3"={"Position"={"x"=365.49564, "y"=408.5937, "z"=0.9895617}, "UV"={"u"=0.0, "v"=0.0}, "Colour"=12517256}, "Alpha"=0.0, "Alpha Blending Enabled"=FALSE, "Colour"=10145390}, {"Vertex 1"={"Position"={"x"=400.0, "y"=442.25943, "z"=0.98947006}, "UV"={"u"=0.0, "v"=0.0}, "Colour"=12517256}, "Vertex 2"={"Position"={"x"=400.0, "y"=434.1526, "z"=0.9895892}, "UV"={"u"=0.0, "v"=0.0}, "Colour"=12517256}, "Vertex 3"={"Position"={"x"=396.07202, "y"=434.0735, "z"=0.9895953}, "UV"={"u"=0.0, "v"=0.0}, "Colour"=12517256}, "Alpha"=0.0, "Alpha Blending Enabled"=FALSE, "Colour"=658951}, {"Vertex 1"={"Position"={"x"=502.10248, "y"=399.48126, "z"=0.9893889}, "UV"={"u"=0.0, "v"=0.0}, "Colour"=12517256}, "Vertex 2"={"Position"={"x"=485.95386, "y"=401.00818, "z"=0.9894933}, "UV"={"u"=0.0, "v"=0.0}, "Colour"=12517256}, "Vertex 3"={"Position"={"x"=486.98724, "y"=398.35367, "z"=0.9897707}, "UV"={"u"=0.0, "v"=0.0}, "Colour"=12517256}, "Alpha"=0.0, "Alpha Blending Enabled"=FALSE, "Colour"=9091426}, {"Vertex 1"={"Position"={"x"=407.6209, "y"=433.84442, "z"=0.9896132}, "UV"={"u"=0.0, "v"=0.0}, "Colour"=12517256}, "Vertex 2"={"Position"={"x"=409.59305, "y"=441.8486, "z"=0.98950064}, "UV"={"u"=0.0, "v"=0.0}, "Colour"=12517256}, "Vertex 3"={"Position"={"x"=413.86533, "y"=441.3613, "z"=0.9895369}, "UV"={"u"=0.0, "v"=0.0}, "Colour"=12517256}, "Alpha"=0.0, "Alpha Blending Enabled"=FALSE, "Colour"=131842}, {"Vertex 1"={"Position"={"x"=299.14365, "y"=127.179695, "z"=0.98972636}, "UV"={"u"=0.0, "v"=0.0}, "Colour"=12517256}, "Vertex 2"={"Position"={"x"=278.11005, "y"=127.45417, "z"=0.9896591}, "UV"={"u"=0.0, "v"=0.0}, "Colour"=12517256}, "Vertex 3"={"Position"={"x"=278.23944, "y"=120.85737, "z"=0.98926175}, "UV"={"u"=0.0, "v"=0.0}, "Colour"=12517256}, "Alpha"=0.0, "Alpha Blending Enabled"=FALSE, "Colour"=131841}, {"Vertex 1"={"Position"={"x"=417.69724, "y"=440.7109, "z"=0.9895852}, "UV"={"u"=0.0, "v"=0.0}, "Colour"=12517256}, "Vertex 2"={"Position"={"x"=421.20996, "y"=448.31607, "z"=0.98949325}, "UV"={"u"=0.0, "v"=0.0}, "Colour"=12517256}, "Vertex 3"={"Position"={"x"=425.17258, "y"=447.3146, "z"=0.98956454}, "UV"={"u"=0.0, "v"=0.0}, "Colour"=12517256}, "Alpha"=0.0, "Alpha Blending Enabled"=FALSE, "Colour"=131841}, {"Vertex 1"={"Position"={"x"=696.25714, "y"=355.18262, "z"=0.98958987}, "UV"={"u"=0.0, "v"=0.0}, "Colour"=12517256}, "Vertex 2"={"Position"={"x"=690.1191, "y"=337.60867, "z"=0.98951393}, "UV"={"u"=0.0, "v"=0.0}, "Colour"=12517256}, "Vertex 3"={"Position"={"x"=683.931, "y"=340.25684, "z"=0.98953646}, "UV"={"u"=0.0, "v"=0.0}, "Colour"=12517256}, "Alpha"=0.0, "Alpha Blending Enabled"=FALSE, "Colour"=10672756}, {"Vertex 1"={"Position"={"x"=372.1155, "y"=458.98697, "z"=0.9895123}, "UV"={"u"=0.0, "v"=0.0}, "Colour"=12517256}, "Vertex 2"={"Position"={"x"=372.0999, "y"=453.91602, "z"=0.98951197}, "UV"={"u"=0.0, "v"=0.0}, "Colour"=12517256}, "Vertex 3"={"Position"={"x"=368.48776, "y"=452.57986, "z"=0.9896035}, "UV"={"u"=0.0, "v"=0.0}, "Colour"=12517256}, "Alpha"=0.0, "Alpha Blending Enabled"=FALSE, "Colour"=5797439}, {"Vertex 1"={"Position"={"x"=427.9001, "y"=453.91602, "z"=0.98951197}, "UV"={"u"=0.0, "v"=0.0}, "Colour"=12517256}, "Vertex 2"={"Position"={"x"=427.8845, "y"=458.98697, "z"=0.9895123}, "UV"={"u"=0.0, "v"=0.0}, "Colour"=12517256}, "Vertex 3"={"Position"={"x"=431.49448, "y"=457.60767, "z"=0.98960376}, "UV"={"u"=0.0, "v"=0.0}, "Colour"=12517256}, "Alpha"=0.0, "Alpha Blending Enabled"=FALSE, "Colour"=5797439}, {"Vertex 1"={"Position"={"x"=372.1155, "y"=458.98697, "z"=0.9895123}, "UV"={"u"=0.0, "v"=0.0}, "Colour"=12517256}, "Vertex 2"={"Position"={"x"=376.1374, "y"=461.78098, "z"=0.98958975}, "UV"={"u"=0.0, "v"=0.0}, "Colour"=12517256}, "Vertex 3"={"Position"={"x"=379.9003, "y"=462.82288, "z"=0.98952234}, "UV"={"u"=0.0, "v"=0.0}, "Colour"=12517256}, "Alpha"=0.0, "Alpha Blending Enabled"=FALSE, "Colour"=11133561}, {"Vertex 1"={"Position"={"x"=466.43457, "y"=404.58322, "z"=0.98938376}, "UV"={"u"=0.0, "v"=0.0}, "Colour"=12517256}, "Vertex 2"={"Position"={"x"=451.1117, "y"=405.76608, "z"=0.98953724}, "UV"={"u"=0.0, "v"=0.0}, "Colour"=12517256}, "Vertex 3"={"Position"={"x"=453.6991, "y"=404.1098, "z"=0.98970187}, "UV"={"u"=0.0, "v"=0.0}, "Colour"=12517256}, "Alpha"=0.0, "Alpha Blending Enabled"=FALSE, "Colour"=9289061}, {"Vertex 1"={"Position"={"x"=689.1351, "y"=288.03708, "z"=0.9894408}, "UV"={"u"=0.0, "v"=0.0}, "Colour"=12517256}, "Vertex 2"={"Position"={"x"=693.37805, "y"=310.46698, "z"=0.98952615}, "UV"={"u"=0.0, "v"=0.0}, "Colour"=12517256}, "Vertex 3"={"Position"={"x"=693.6034, "y"=307.21713, "z"=0.9896555}, "UV"={"u"=0.0, "v"=0.0}, "Colour"=12517256}, "Alpha"=0.0, "Alpha Blending Enabled"=FALSE, "Colour"=3755049}, {"Vertex 1"={"Position"={"x"=653.6545, "y"=220.1329, "z"=0.989419}, 
